vi "Set Version Independent.vi"(8 "error in (no error)":errorcluster, 10 "versionIndependent":bool, 11 "NI_AB_API_Targetfile in":refnum<class "NI_AB_API_Targetfile.lvclass">) -> (0 "error out":errorcluster, 3 "NI_AB_API_Targetfile out":refnum<class "NI_AB_API_Targetfile.lvclass">)   [LabVIEW 2020, in "NI_AB_API_Targetfile.lvclass"]
uses:
  <vilib>/AppBuilder/AB_API/Targetfile/NI_AB_API_Targetfile.lvclass
  e:/builds/penguin/labview/branches/2020/dev/dist/vi.lib/AppBuilder/AB_API/Build/NI_AB_API_Build.lvclass
  <vilib>/AppBuilder/AB_Classes/TargetFile/AB_Targetfile.lvclass
  e:/builds/penguin/labview/branches/2020/dev/dist/vi.lib/AppBuilder/AB_Classes/Build/AB_Build.lvclass
  <vilib>/AppBuilder/AB_API/Build/NI_AB_API_Build.lvclass
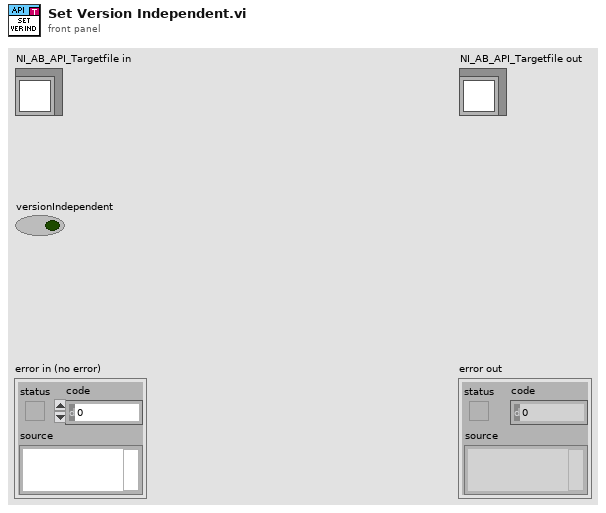
[diagram p1: front panel]
types:
  T1 = typedef "AB_Targetfile.ctl" = cluster{"targetfileName":string, "targetfileGUID":string, "enableDebugging":bool, "versionInfo":cluster{"productName":string, "legalCopyright":string, "companyName":string, "internalName":string, "fileDescription":string}, "eng_consolidatedTypeInfo":string, "fastFileFormat":bool, "eng_LEIFBuildData":u32, "versionIndependent":bool}
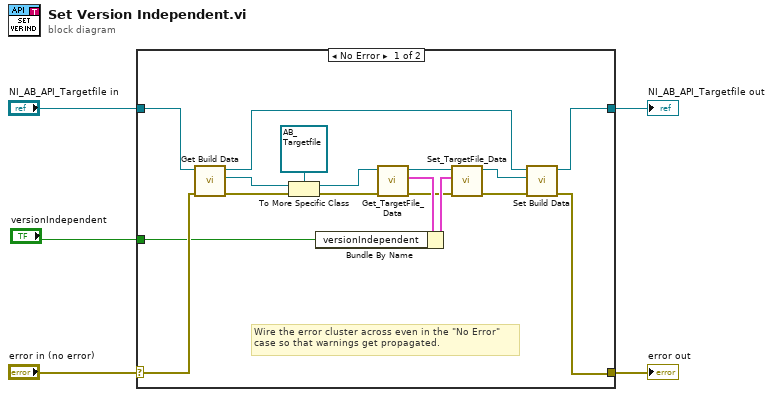
[diagram p0: block diagram]
diagram:
  n1 = case shown="No Error" "error in (no error)" {
    selector: "error in (no error)" -> [w8 w24]
    tunnel: [w7 w24] -> w4
    tunnel: [w9 w23] -> w2
    tunnel: "NI_AB_API_Targetfile in" -> [w10 w23]
    tunnel: "versionIndependent" -> [w6 _]
    frame No Error {
      # "Wire the error cluster across even in the \"No Error\"\ncase so that warnings get propagated."
      n2 = call <vilib>:"Get Build Data.vi"("error in (no error)"=w8, "NI_AB_API_Build in"=w10) -> ("error out"=w15:errorcluster, "AB_Build.lvclass"=w17:refnum<class "AB_Build.lvclass">, "NI_AB_API_Build out"=w19:refnum<class "NI_AB_API_Targetfile.lvclass">)  [unwired: 7 in]
      n3 = To More Specific Class(target class=refnum<class "AB_Targetfile.lvclass"> refnum ("AB_Targetfile in"), reference=w17, error in=w15) -> (specific class reference=w16:refnum<class "AB_Targetfile.lvclass">, error out=w13:errorcluster)
      n4 = call <vilib>:"Get_TargetFile_Data.vi"("error in (no error)"=w13, "AB_Targetfile in"=w16) -> ("error out"=w12:errorcluster, "data"=w21:T1, "AB_Targetfile out"=w22:refnum<class "AB_Targetfile.lvclass">)  [unwired: 7 in]
      n5 = Bundle By Name(cluster=w21, "versionIndependent"=w6) -> (w20:T1)
      n6 = call <vilib>:"Set_TargetFile_Data.vi"("error in (no error)"=w12, "data"=w20, "AB_Targetfile in"=w22) -> ("error out"=w11:errorcluster, "AB_Targetfile out"=w14:refnum<class "AB_Targetfile.lvclass">)  [unwired: 7 in]
      n7 = call <vilib>:"Set Build Data.vi"("error in (no error)"=w11, "AB_Build.lvclass"=w14, "NI_AB_API_Build in"=w19) -> ("error out"=w7:errorcluster, "NI_AB_API_Build out"=w9:refnum<class "NI_AB_API_Targetfile.lvclass">)  [unwired: 7 in]
    }
    frame Error {
    }
  }
  "error out" <- w4
  "NI_AB_API_Targetfile out" <- w2
